vi "Simple Add.vi"(9 "y 2":dbl, 10 "y":dbl, 11 "x":dbl) -> (3 "x+y":dbl)   [LabVIEW 2016]
panel:
  in  "Boolean":bool
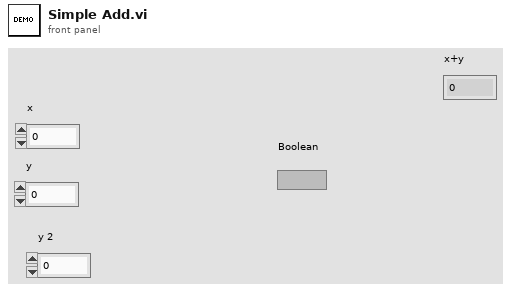
[diagram p1: front panel]
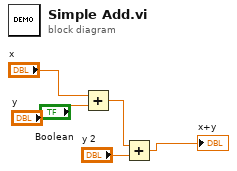
[diagram p0: block diagram]
diagram:
  n1 = Add(x="x", y="y") -> (x+y=w3:dbl)
  n2 = Add(x=w3, y="y 2") -> (x+y=→"x+y":dbl)
